vi "sepios_pressureSensor_old.vi"() -> ()   [LabVIEW 2013]
uses:
  <vilib>/myRIO/Instrument Drivers/Utilities/Utilities.lvlib
panel:
  in  "Tab Control":enum32{"User", "Tuning"}(tab)
  out "Depth [m]":dbl
  out "Depth":cluster{dbl, "Depth [m]":dbl}(graph)
  out "Pressure [Bar]":dbl
  out "P_ref [Pa]":dbl
  in  "Calibrate":bool
  in  "Waterdensity":dbl=1000.0
  in  "Max. Depth":dbl=5.0
  out "error out":errorcluster
  in  "Stop Button":bool
  # "Pressure Sensor MPX4250A"
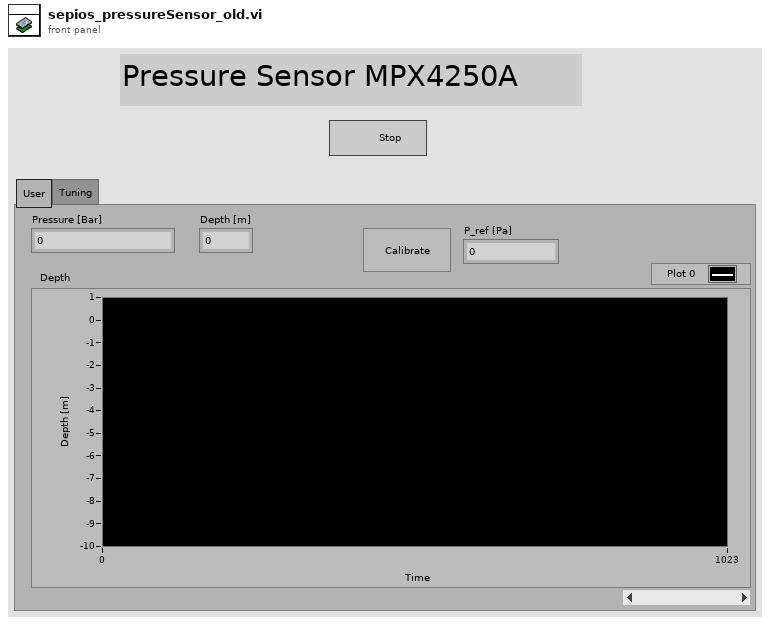
[diagram p1: front panel]
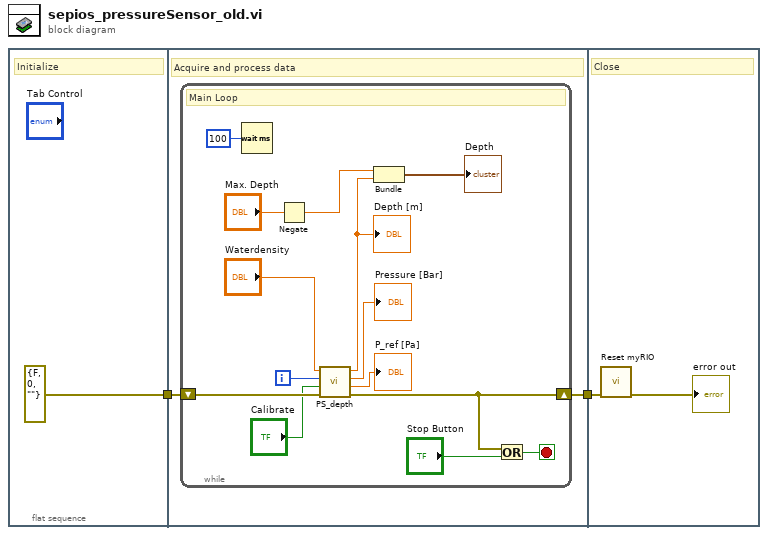
[diagram p0: block diagram]
diagram:
  n1 = flat-sequence {
    tunnel: [errorcluster {"status"=FALSE, "code"=0, "source"=""} ("error out")] -> w2
    tunnel: w2 -> [w5]
    tunnel: [w4] -> w1
    tunnel: w1 -> [w21]
    frame #0 {
      # "Initialize"
    }
    frame #1 {
      # "Acquire and process data"
      n2 = while {
        shift-right: [w15] -> w4
        shift-left: w5 -> [w17]
        i -> [w14]
        stop <- w18 stop-if-true
        # "Main Loop"
        n3 = Wait (ms)(milliseconds to wait=u32 100) -> ()  [unwired: 1 out]
        n4 = Negate(x="Max. Depth") -> (-x=w6:dbl)
        n5 = call "PS_depth.vi"("error in (no error)"=w17, "Calibrate"="Calibrate", "Loop Index"=w14, "Water density [kg/m^3]"="Waterdensity") -> ("error out"=w15:errorcluster, "P_ref [Pa]"=→"P_ref [Pa]":dbl, "Pressure [Bar]"=→"Pressure [Bar]":dbl, "Depth [m]"=w10:dbl)
        "Depth [m]" <- w10
        n6 = Bundle(w6, "Depth [m]"=w10) -> (→"Depth":cluster{dbl, "Depth [m]":dbl})  [unwired: 1 in]
        n7 = Or(x=w15, y="Stop Button") -> (x .or. y?=w18:bool)
      }
    }
    frame #2 {
      # "Close"
      n8 = call <vilib>:"Reset myRIO.vi"("error in (no error)"=w21) -> ("error out"=→"error out":errorcluster)  [unwired: 10 in]
    }
  }
